vi "MultiCha-TransmitReceive.vi"() -> ()   [LabVIEW 2023]
uses:
  <instrlib>/BTICardLib/Private/Initialize By Card Number and Core Number.vi
  <instrlib>/BTICardLib/Private/Configure Core From XML.vi
  <instrlib>/BTI429Lib/Private/Tx/Configure/Configure Tx Channel From XML.vi
  <instrlib>/BTI429Lib/Private/Rx/Configure/Configure Rx Channel From XML.vi
  <instrlib>/BTI429Lib/Private/Rx/Configure/Get Rx Label Handle Name.vi
  <instrlib>/BTI429Lib/Private/Core/Action-Status/Start All Channels.vi
  <instrlib>/BTI429Lib/Private/Utility/Get BNR Mantissa.vi
  <instrlib>/BTI429Lib/Private/Core/Action-Status/Stop All Channels.vi
  <instrlib>/BTICardLib/BTICardLV.lvlib
  <instrlib>/BTI429Lib/BTI429LV.lvlib
panel:
  out "mantissa out":u32 format="%08x"
  out "value":u32 format="%08x"
  in  "stop":bool
  out "error out":errorcluster
  in  "Rx channel number":i32=3
  out "Channel Rx Xml Path":path
  in  "Channel Configuration Rx XML file name":string="Channel Config.xml"
  in  "Tx channel number":i32=18
  out "Core Xml Path":path
  out "Channel Tx Xml Path":path
  in  "Core Configuration XML file name":string="Core Config.xml"
  in  "Channel ConfigurationTx XML file name":string="Channel Config.xml"
  in  "core number":i32
  in  "card number":i32
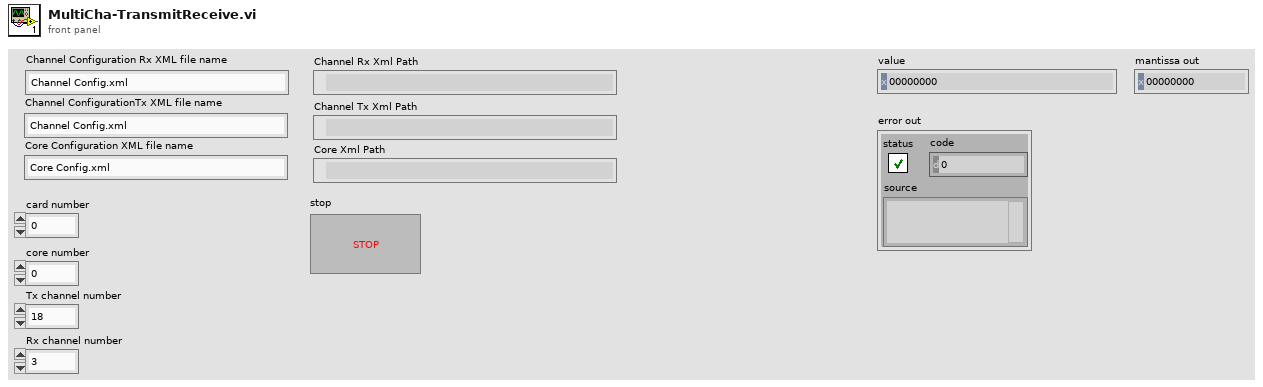
[diagram p1: front panel]
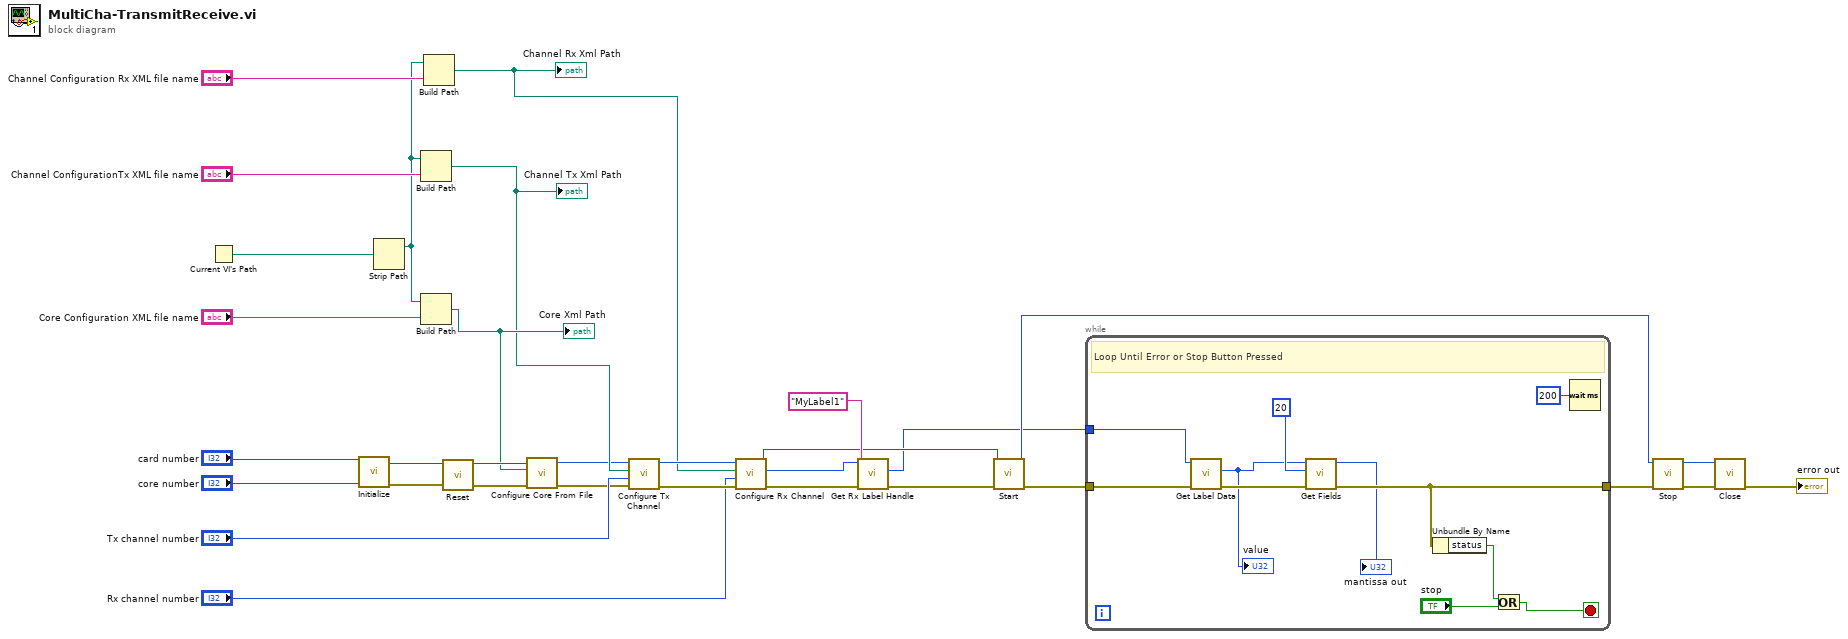
[diagram p0: block diagram]
diagram:
  n1 = Current VI's Path() -> (path=w27:path)
  n2 = call-poly <instrlib>:"Initialize.vi"("core number"="core number", "card number"="card number") -> ("error out"=w29:errorcluster, "core handle out"=w30:u64)  [unwired: 8 in]
  n3 = Strip Path(path=w27) -> (stripped path=w16:path)  [unwired: 1 out]
  n4 = Build Path(base path=w16, name or relative path="Channel ConfigurationTx XML file name") -> (appended path=w23:path)
  "Channel Tx Xml Path" <- w23
  n5 = Build Path(base path=w16, name or relative path="Core Configuration XML file name") -> (appended path=w24:path)
  "Core Xml Path" <- w24
  n6 = Build Path(base path=w16, name or relative path="Channel Configuration Rx XML file name") -> (appended path=w15:path)
  "Channel Rx Xml Path" <- w15
  n7 = call <instrlib>:"Reset.vi"("error in (no error)"=w29, "core handle in"=w30) -> ("error out"=w20:errorcluster, "core handle out"=w28:u64)  [unwired: 8 in]
  n8 = call-poly <instrlib>:"Configure Core From File.vi"("error in (no error)"=w20, "configuration file path"=w24, "core handle in"=w28) -> ("error out"=w19:errorcluster, "core handle out"=w22:u64)  [unwired: 7 in]
  n9 = call-poly <instrlib>:"Configure Tx Channel.vi"("error in (no error)"=w19, "channel number in"="Tx channel number", "configuration file path"=w23, "core handle in"=w22) -> ("error out"=w14:errorcluster, "core handle out"=w18:u64)  [unwired: 5 in, 1 out]
  n10 = call-poly <instrlib>:"Configure Rx Channel.vi"("error in (no error)"=w14, "channel number in"="Rx channel number", "configuration file path"=w15, "core handle in"=w18) -> ("error out"=w11:errorcluster, "channel handle out"=w12:u64, "core handle out"=w5:u64)  [unwired: 5 in]
  n11 = call-poly <instrlib>:"Get Rx Label Handle.vi"("error in (no error)"=w11, "label name"="MyLabel1", "channel handle in"=w12) -> ("error out"=w4:errorcluster, "label handle out"=w3:u64)  [unwired: 6 in, 1 out]
  n12 = call-poly <instrlib>:"Start.vi"("error in (no error)"=w4, "core handle in"=w5) -> ("error out"=w2:errorcluster, "core handle out"=w9:u64)  [unwired: 8 in]
  n13 = while {
    tunnel: w3 -> [w40]
    tunnel: w2 -> [w41]
    tunnel: [w34] -> w1
    stop <- w43 stop-if-true
    # "Loop Until Error or Stop Button Pressed"
    n14 = call <instrlib>:"Get Label Data.vi"("error in (no error)"=w41, "label handle in"=w40) -> ("error out"=w36:errorcluster, "value"=w35:u32)  [unwired: 7 in, 1 out]
    "value" <- w35
    n15 = call-poly <instrlib>:"Get Fields.vi"("error in (no error)"=w36, "significant digits"=u16 20 ("most significant bit"), "message"=w35) -> ("error out"=w34:errorcluster, "mantissa out"=→"mantissa out":u32)  [unwired: 7 in]
    n16 = Unbundle By Name(w34) -> ("status"=w39:bool)
    n17 = Or(x=w39, y="stop") -> (x .or. y?=w43:bool)
    n18 = Wait (ms)(milliseconds to wait=u32 200) -> ()  [unwired: 1 out]
  }
  n19 = call-poly <instrlib>:"Stop.vi"("error in (no error)"=w1, "core handle in"=w9) -> ("error out"=w7:errorcluster, "core handle out"=w8:u64)  [unwired: 8 in]
  n20 = call <instrlib>:"Close.vi"("error in (no error)"=w7, "core handle in"=w8) -> ("error out"=→"error out":errorcluster)  [unwired: 8 in, 1 out]
